vi "Helm Waveforms.vi"(10 "Log Data In":cluster{refnum<class "RDS State.lvclass">[]}[](array[cluster]), 11 "Log Header In":T1) -> (2 "Log Data Out":cluster{refnum<class "RDS State.lvclass">[]}[](array[cluster]), 3 "Log Header Out":T1, 5 "Heading Command":waveform(dbl)[](array[waveform]))   [LabVIEW 2015, in "Log Waveform Processors.lvlib"]
uses:
  Log Waveform Processors.lvlib
  RDS State Tracker/RDS State/RDS State.lvclass
  Actors/RDS Logger Actor/RDS Logger Actor/RDS Logger Actor/Logger Header.ctl
  RDS State Tracker/RDS State/RDS State.lvclass/RDS State.ctl
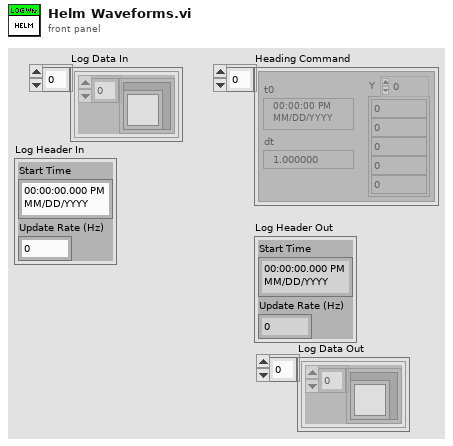
[diagram p1: front panel]
types:
  T1 = typedef "Log Waveform Processors.lvlib/Logger Header.ctl" = cluster{"Start Time":timestamp, "Update Rate (Hz)":dbl}
  T2 = typedef "RDS Child Messages.lvlib/Helm Status Control.ctl" = cluster{"Helm State":T3, "Heading Command Control":T4, "Steering Command Control":T5, "Last Command Time":timestamp, "Gains":T6, "Current Heading":dbl, "Port Throttle":i16, "STBD Throttle":i16, "Limiter":dbl}
  T3 = typedef "RDS Helm Actor.lvlib/Helm State.ctl" = enum16{"Idle", "Executing Heading Command", "Executing Steering Command"}
  T4 = typedef "RDS Child Messages.lvlib/Heading Command Cntrl.ctl" = cluster{"Throttle":i16, "Heading":sgl, "Duration (s)":i16}
  T5 = typedef "RDS Child Messages.lvlib/Steering Command Cntrl.ctl" = cluster{"Throttle":i16, "Rudder":i8, "Duration (s)":u16}
  T6 = typedef "RDS Child Messages.lvlib/PID Gains Control.ctl" = cluster{"P (Kc)":sgl, "I (Ti)":sgl, "D (Td)":sgl}
  T7 = typedef "RDS Libraries.lvlib/NMEA.lvlib/NMEA_GPRMC-data.ctl" = cluster{"TimeStamp":timestamp, "Validity":bool, "Latitude":dbl, "Latitude-Direction":T8, "Longitude":dbl, "Longitude-Direction":T9, "Speed in knots":sgl, "True course":sgl, "Date Stamp":timestamp, "Magnetic Variation (East/West)":sgl, "GPS Latitude":dbl, "GPS Longitude":dbl}
  T8 = typedef "RDS Libraries.lvlib/NMEA.lvlib/NMEA_LatitudeDirection.ctl" = enum16{"", "North", "South"}
  T9 = typedef "RDS Libraries.lvlib/NMEA.lvlib/NMEA_LongitudeDirection.ctl" = enum16{"", "East", "West"}
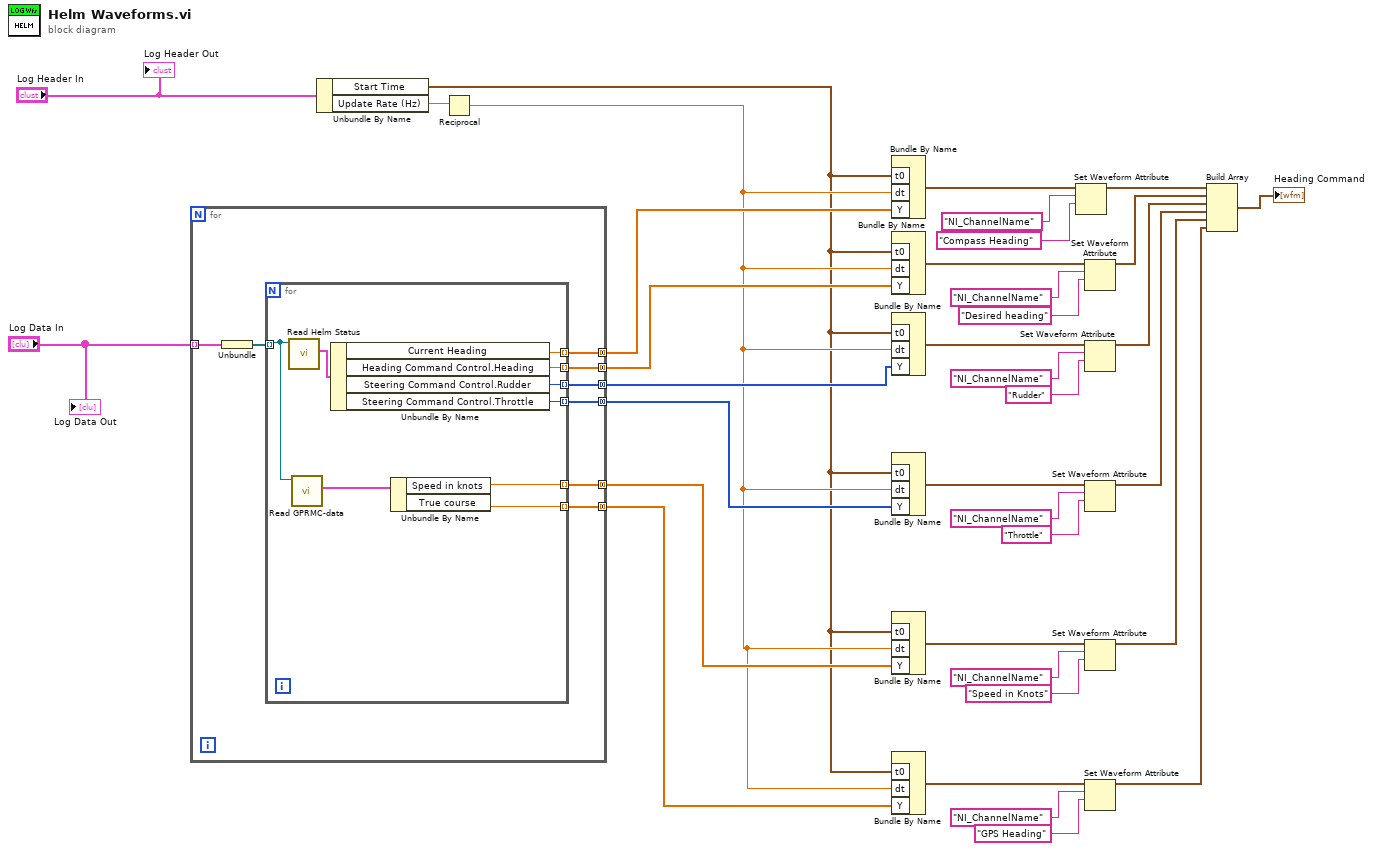
[diagram p0: block diagram]
diagram:
  n1 = for {
    tunnel: "Log Data In" -> [w44] mode=indexing
    tunnel: [w42] -> w20 mode=concatenating
    tunnel: [w41] -> w19 mode=concatenating
    tunnel: [w40] -> w6 mode=concatenating
    tunnel: [w39] -> w4 mode=concatenating
    tunnel: [w38] -> w8 mode=concatenating
    tunnel: [w37] -> w7 mode=concatenating
    n2 = Unbundle(w44) -> (w43:refnum<class "RDS State.lvclass">[])
    n3 = for {
      tunnel: w43 -> [w50] mode=indexing
      tunnel: [w52] -> w42 mode=indexing
      tunnel: [w51] -> w41 mode=indexing
      tunnel: [w49] -> w40 mode=indexing
      tunnel: [w48] -> w39 mode=indexing
      tunnel: [w47] -> w38 mode=indexing
      tunnel: [w46] -> w37 mode=indexing
      n4 = call "Read Helm Status.vi"("RDS State in"=w50) -> ("Helm Status"=w53:T2)  [unwired: 8 in, 2 out]
      n5 = call "Read GPRMC-data.vi"("RDS State in"=w50) -> ("GPRMC-data"=w45:T7)  [unwired: 8 in, 2 out]
      n6 = Unbundle By Name(w53) -> ("Current Heading"=w52:dbl, "Heading Command Control.Heading"=w51:sgl, "Steering Command Control.Rudder"=w47:i8, "Steering Command Control.Throttle"=w46:i16)
      n7 = Unbundle By Name(w45) -> ("Speed in knots"=w49:sgl, "True course"=w48:sgl)
    }
  }
  n8 = Unbundle By Name("Log Header In") -> ("Start Time"=w3:timestamp, "Update Rate (Hz)"=w21:dbl)
  n9 = Reciprocal(x=w21) -> (1/x=w5:dbl)
  n10 = Bundle By Name("t0"=w3, "dt"=w5, "Y"=w20) -> (w24:waveform(dbl))  [unwired: 1 in]
  n11 = Bundle By Name("t0"=w3, "dt"=w5, "Y"=w19) -> (w26:waveform(sgl))  [unwired: 1 in]
  n12 = Bundle By Name("t0"=w3, "dt"=w5, "Y"=w8) -> (w27:waveform(i8))  [unwired: 1 in]
  n13 = Bundle By Name("t0"=w3, "dt"=w5, "Y"=w7) -> (w18:waveform(i16))  [unwired: 1 in]
  n14 = Bundle By Name("t0"=w3, "dt"=w5, "Y"=w6) -> (w11:waveform(sgl))  [unwired: 1 in]
  n15 = Bundle By Name("t0"=w3, "dt"=w5, "Y"=w4) -> (w12:waveform(sgl))  [unwired: 1 in]
  n16 = Set Waveform Attribute(5:"Compass Heading" ("name"), 6:"NI_ChannelName" ("name"), 7:w24) -> (3:w28:waveform(dbl))  [unwired: 1 in, 2 out]
  n17 = Set Waveform Attribute(5:"Desired heading" ("name"), 6:"NI_ChannelName" ("name"), 7:w26) -> (3:w29:waveform(sgl))  [unwired: 1 in, 2 out]
  n18 = Set Waveform Attribute(5:"Rudder" ("name"), 6:"NI_ChannelName" ("name"), 7:w27) -> (3:w30:waveform(i8))  [unwired: 1 in, 2 out]
  n19 = Set Waveform Attribute(5:"Throttle" ("name"), 6:"NI_ChannelName" ("name"), 7:w18) -> (3:w15:waveform(i16))  [unwired: 1 in, 2 out]
  n20 = Set Waveform Attribute(5:"Speed in Knots" ("name"), 6:"NI_ChannelName" ("name"), 7:w11) -> (3:w2:waveform(sgl))  [unwired: 1 in, 2 out]
  n21 = Set Waveform Attribute(5:"GPS Heading" ("name"), 6:"NI_ChannelName" ("name"), 7:w12) -> (3:w1:waveform(sgl))  [unwired: 1 in, 2 out]
  n22 = Build Array(w28, w29, w30, w15, w2, w1) -> (→"Heading Command":waveform(dbl)[])
  "Log Header Out" <- "Log Header In"
  "Log Data Out" <- "Log Data In"
